vi "remove channel from configuration.vi"(5 "channels":refnum<vi>, 7 "user event":T1, 8 "error in":errorcluster, 9 "channels value":i32, 10 "engine configuration in":refnum<class "engine configuration.lvclass">, 11 "Scan Engine configuration in":refnum<class "Scan Engine configuration.lvclass">) -> (0 "error out":errorcluster, 2 "engine configuration out":refnum<class "engine configuration.lvclass">, 3 "Scan Engine configuration out":refnum<class "Scan Engine configuration.lvclass">)   [LabVIEW 2013, in "Scan Engine editor node.lvclass"]
uses:
  Scan Engine editor node.lvclass
  <vilib>/NI/Module Execution Interface/Engine Configuration/engine configuration.lvclass
  module/configuration/Scan Engine configuration.lvclass
  <vilib>/NI/Configuration Framework/Node/UserEventRef.ctl
  <vilib>/NI/Configuration Framework/Controls/EventCluster.ctl
  <vilib>/NI/Configuration Framework/serializable configuration/NISE_CEF_serializable configuration.lvclass/NISE_CEF_serializable configuration.ctl
  <vilib>/NI/Configuration Framework/serializable configuration/NISE_CEF_serializable configuration.lvclass
  <vilib>/NI/Configuration Framework/NISE_CEF_TreeControl.lvlib
  <vilib>/NI/Configuration Framework/Node/NISE_CEF_Node.lvclass
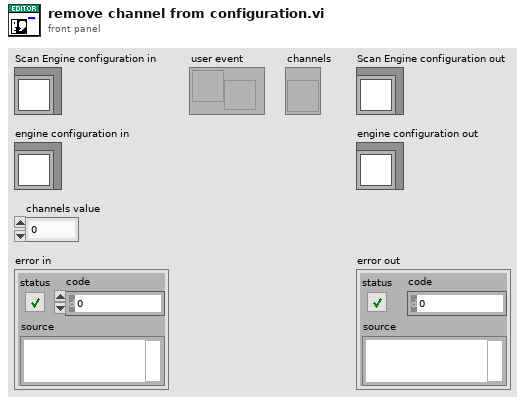
[diagram p1: front panel]
types:
  T1 = typedef "NISE_CEF_Node.lvclass/UserEventRef.ctl" = refnum<user-event>
  T2 = typedef "Scan Engine editor node.lvclass/table line.ctl" = cluster{"tag":string, "channel":refnum<class "TBM channel.lvclass">}
  T3 = typedef "NISE_CEF_TreeControl.lvlib/EventCluster.ctl" = cluster{"command":string, "data":string}
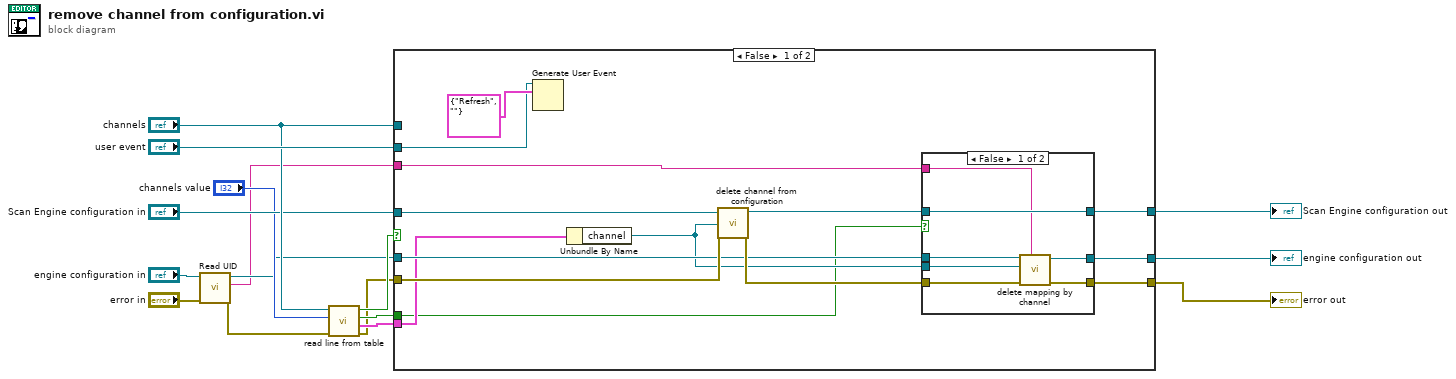
[diagram p0: block diagram]
diagram:
  n1 = call <vilib>:"Read UID.vi"("error in"="error in", "configuration in"="engine configuration in") -> ("error out"=w4:errorcluster, "instance id"=w1:string, "configuration out"=w2:refnum<class "engine configuration.lvclass">)  [unwired: 7 in]
  n2 = call "read line from table.vi"("error in"=w4, "line number"="channels value", "operations table"="channels") -> ("error out"=w7:errorcluster, "line"=w10:T2, "empty tag?"=w12:bool, "empty channel?"=w11:bool)  [unwired: 5 in]
  n3 = case shown="False" w11 {
    tunnel: w7 -> [w29 w41]
    tunnel: "Scan Engine configuration in" -> [w28 w43]
    tunnel: w2 -> [w27 w42]
    tunnel: [w26 w42] -> w16
    tunnel: [w21 w43] -> w15
    tunnel: [w25 w41] -> w9
    tunnel: w10 -> [w24 _]
    tunnel: w1 -> [w23 _]
    tunnel: w12 -> [w19 _]
    tunnel: "channels" -> [_ _]
    tunnel: "user event" -> [w17 _]
    frame False {
      n4 = Generate User Event(user event=w17, event data cluster=T3 {"command"="Refresh", "data"=""} ("event data")) -> ()  [unwired: 2 in, 2 out]
      n5 = Unbundle By Name(w24) -> ("channel"=w22:refnum<class "TBM channel.lvclass">)
      n6 = call "delete channel from configuration.vi"("error in"=w29, "channel"=w22, "Scan Engine configuration in"=w28) -> ("error out"=w30:errorcluster, "Scan Engine configuration out"=w20:refnum<class "Scan Engine configuration.lvclass">)  [unwired: 7 in]
      n7 = case shown="False" w19 {
        tunnel: w30 -> [w37 w38]
        tunnel: w27 -> [w36 w40]
        tunnel: [w35 w40] -> w26
        tunnel: [w34 w38] -> w25
        tunnel: w23 -> [w31 _]
        tunnel: w22 -> [w33 _]
        tunnel: [w32 w39] -> w21
        tunnel: w20 -> [w32 w39]
        frame False {
          n8 = call <vilib>:"delete mapping by channel.vi"("owner ID"=w31, "error in"=w37, "channel"=w33, "engine configuration in"=w36) -> ("error out"=w34:errorcluster, "engine configuration out"=w35:refnum<class "engine configuration.lvclass">)  [unwired: 6 in]
        }
        frame True {
        }
      }
    }
    frame True {
    }
  }
  "engine configuration out" <- w16
  "Scan Engine configuration out" <- w15
  "error out" <- w9
